vi "TEST Variant to string.vi"(7 "Anything":variant, 11 "error in (no error)":errorcluster) -> (8 "String Value":string, 15 "error out":errorcluster)   [LabVIEW 2011]
doc: "Use in the same way as Read key. Anything in may contain a cluster.\nAny data wired to Anything must be named, that includes any item in a cluster.\nThis is a slow VI, keep in mind when desiding where to use.\n\nARRAY SUPPIORT FUNKER IKKE. \n\nThe cluster can contain anything(Including other clusters) except:\nARRAY\nVariant\nPicture\nTag\nWaveform\nDigital Waveform\nDigital Data\nExpressData\nRefnum\nExternal Data\nVI\nPoly VI\nLabview Class Instance\nFixed point\n\nOn Error: No operation"
uses:
  emi Lib/Basic/0 - General/Error/emi_Create Error.vi
  <vilib>/Utility/VariantDataType/GetNumericInfo.vi
  <vilib>/Utility/VariantDataType/VariantType.lvlib
panel:
  in  "String":string
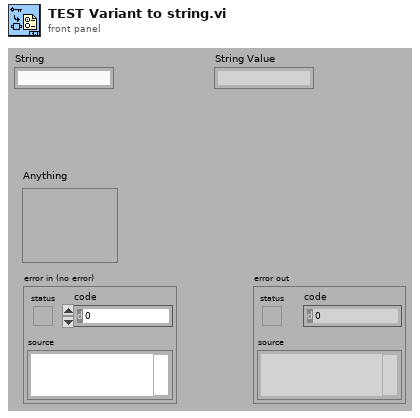
[diagram p1: front panel]
types:
  T1 = typedef "VariantType.lvlib/Type.ctl" = enum8{"Invalid Type", "Void", "I8", "I16", "I32", "I64", "U8", "U16", "U32", "U64", "Single Float", "Double Float", "Extended Float", "Single Complex", "Double Complex", "Extended Complex", "Enum U8", "Enum U16", "Enum U32", "Enum U64", "Single Float With Unit", "Double Float With Unit", "Extended Float With Unit", "Single Complex with Unit", "Double Complex with Unit", "Extended Complex with Unit", "Boolean", "String", "Path", "Picture", "Tag", "Array", "Cluster", "Variant", "LV Variant", "Waveform", "Timestamp", "Digital Waveform", "Digital Data", "ExpressData", "Refnum", "External Data", "VI", "Poly VI", "LabVIEW Class Instance", "Fixed Point"}
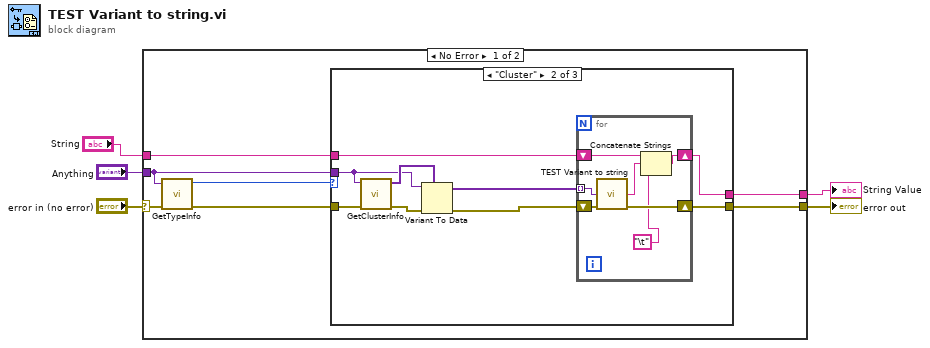
[diagram p0: block diagram]
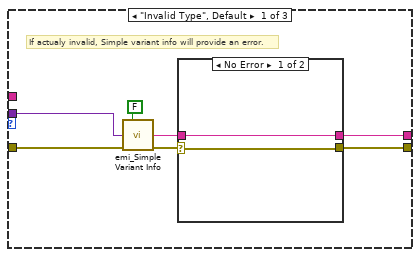
[diagram p2: hidden frame]
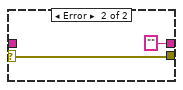
[diagram p3: hidden frame]
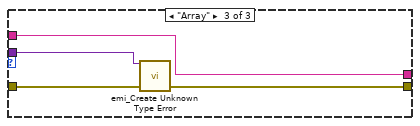
[diagram p4: hidden frame]
diagram:
  n1 = case shown="No Error" "error in (no error)" {
    selector: "error in (no error)" -> [w9 w45]
    tunnel: "Anything" -> [w11 _]
    tunnel: [w8 w45] -> w3
    tunnel: [w7 w44] -> w2
    tunnel: "String" -> [w6 w44]
    frame No Error {
      n2 = call <vilib>:"GetTypeInfo.vi"("error in (no error)"=w9, "Variant"=w11) -> ("error out"=w10:errorcluster, "Type Enum"=w12:T1)  [unwired: 5 in, 3 out]
      n3 = case shown="\"Cluster\"" w12 {
        tunnel: w11 -> [w19 w27 w41]
        tunnel: w10 -> [w18 w31 w42]
        tunnel: [w17 w32 w43] -> w8
        tunnel: [w13 w25 w40] -> w7
        tunnel: w6 -> [_ w24 w40]
        frame "Invalid Type", Default {
          # "If actualy invalid, Simple variant info will provide an error."
          n4 = call "emi_Simple Variant Info.vi"("use system decimal point (T)"=FALSE, "Anything"=w19, "error in(no error)"=w18) -> ("String Value"=w16:string, "error out"=w15:errorcluster)  [unwired: 9 in, 2 out]
          n5 = case shown="No Error" w15 {
            selector: w15 -> [w20 w23]
            tunnel: [w20 w23] -> w17
            tunnel: w16 -> [w21 _]
            tunnel: [w21 "" ("String Value")] -> w13
            frame No Error {
            }
            frame Error {
            }
          }
        }
        frame "Cluster" {
          n6 = call <vilib>:"GetClusterInfo.vi"("error in (no error)"=w31, "Variant"=w27) -> ("error out"=w30:errorcluster, "Cluster Elements"=w28:variant[])  [unwired: 8 in]
          n7 = Variant To Data(error in=w30, type=w28, Variant=w27) -> (data=w26:variant[], error out=w29:errorcluster)
          n8 = for {
            tunnel: w26 -> [w37] mode=indexing
            shift-right: [w38] -> w32
            shift-left: w29 -> [w39]
            shift-right: [w35] -> w25
            shift-left: w24 -> [w34]
            n9 = call "TEST Variant to string.vi"("Anything"=w37, "error in (no error)"=w39) -> ("String Value"=w36:string, "error out"=w38:errorcluster)  [unwired: 12 in]
            n10 = Concatenate Strings(w34, w36, "\t") -> (w35:string)
          }
        }
        frame "Array" {
          n11 = call "emi_Create Unknown Type Error.vi"("Anything"=w41, "error IO"=w42) -> ("error out"=w43:errorcluster)  [unwired: 13 in]
        }
      }
    }
    frame Error {
    }
  }
  "error out" <- w3
  "String Value" <- w2
